vi "Start Measurements Command.vi"(6 "Reply to me":refnum<class "Result Reply Msg.lvclass">, 8 "error in (no error)":errorcluster, 9 "Objects":string[](array[string]), 10 "Controller name":string="Monitor Controller", 11 "Monitor-Pulse in":refnum<class "Monitor-Pulse.lvclass">) -> (0 "error out":errorcluster, 3 "Monitor-Pulse out":refnum<class "Monitor-Pulse.lvclass">)   [LabVIEW 2016, in "Monitor-Pulse.lvclass"]
uses:
  Monitor-Pulse.lvclass
  C:/Program Files/National Instruments/LabVIEW 2016/vi.lib/ActorFramework/Actor/Actor.lvclass
  Measure_core/Template Module Messages/Result Reply Msg/Result Reply Msg.lvclass
  C:/github/Measure_core/Da Base Messages/Self-Addressed Msg/Self-addressed Msg.lvclass
  <vilib>/ActorFramework/Actor/Actor.lvclass/Actor.ctl
  <vilib>/ActorFramework/Message Enqueuer/Message Enqueuer.lvclass/Message Enqueuer.ctl
  Measure_core/Template Module Messages/Self-Addressed Msg/Self-addressed Msg.lvclass/Self-addressed Msg.ctl
  Measure_core/Controllers/Process Controller Messages/Start Measurements Msg/Start Measurements Msg.lvclass/Start Measurements Msg.ctl
  Measure_core/Template Module Messages/Self-Addressed Msg/Write Return Enqueuer.vi
  <vilib>/ActorFramework/Message Enqueuer/Init from Existing Queue.vi
  <vilib>/ActorFramework/Message Enqueuer/Enqueue.vi
  Measure_core/Controllers/Process Controller Messages/Start Measurements Msg/Start Measurements Msg.lvclass
  C:/Program Files/National Instruments/LabVIEW 2016/vi.lib/ActorFramework/Message/Message.lvclass
  <vilib>/ActorFramework/Message Priority Queue/Priority Enqueue.vi
  <vilib>/ActorFramework/Message Enqueuer/Message Enqueuer.lvclass
  <vilib>/ActorFramework/Actor/Actor.lvclass
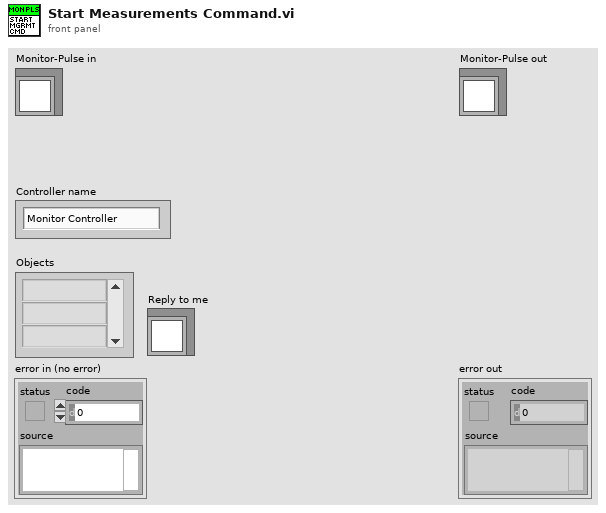
[diagram p1: front panel]
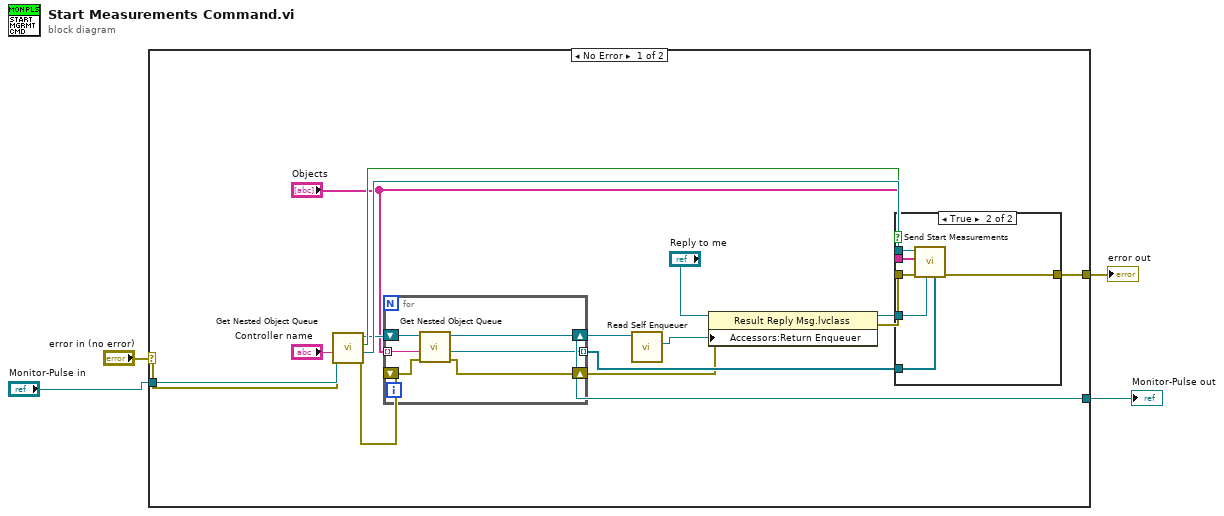
[diagram p0: block diagram]
diagram:
  n1 = case shown="No Error" "error in (no error)" {
    selector: "error in (no error)" -> [w15 w35]
    tunnel: [w17 w35] -> w2
    tunnel: [w5 w34] -> w1
    tunnel: "Monitor-Pulse in" -> [w16 w34]
    frame No Error {
      n2 = call-dynamic "Get Nested Object Queue.vi"("error in (no error)"=w15, "Name"="Controller name", "Measure Object in"=w16) -> ("error out"=w10:errorcluster, "Object Enqueuer"=w19:refnum<class "Message Enqueuer.lvclass">, "Found?"=w18:bool, "Measure Object out"=w11:refnum<class "Monitor-Pulse.lvclass">)  [unwired: 5 in]
      n3 = for {
        tunnel: "Objects" -> [w26] mode=indexing
        shift-right: [w24] -> w5
        shift-left: w11 -> [w25]
        shift-right: [w22] -> w6
        shift-left: w10 -> [w23]
        tunnel: [w21] -> w9 mode=indexing
        n4 = call-dynamic "Get Nested Object Queue.vi"("error in (no error)"=w23, "Name"=w26, "Measure Object in"=w25) -> ("error out"=w22:errorcluster, "Object Enqueuer"=w21:refnum<class "Message Enqueuer.lvclass">, "Measure Object out"=w24:refnum<class "Monitor-Pulse.lvclass">)  [unwired: 5 in, 1 out]
      }
      n5 = call <vilib>:"Read Self Enqueuer.vi"("Actor"=w5) -> ("Self Enqueuer"=w14:refnum<class "Message Enqueuer.lvclass">)  [unwired: 10 in]
      n6 = property class="Result Reply Msg.lvclass"(reference="Reply to me", error in=w6, "Accessors:Return Enqueuer"=w14) -> (reference out=w13:refnum<class "Result Reply Msg.lvclass">, error out=w12:errorcluster)
      n7 = case shown="True" w18 {
        tunnel: w19 -> [_ w33]
        tunnel: w12 -> [w27 w32]
        tunnel: [w27 w31] -> w17
        tunnel: w13 -> [_ w30]
        tunnel: w9 -> [_ w29]
        tunnel: "Objects" -> [_ w28]
        frame False {
        }
        frame True {
          n8 = call "Send Start Measurements.vi"("Objects enqueuers"=w29, "Reply to"=w30, "error in (no error)"=w32, "Objects"=w28, "Message Enqueuer"=w33) -> ("error out"=w31:errorcluster)  [unwired: 5 in, 1 out]
        }
      }
    }
    frame Error {
    }
  }
  "error out" <- w2
  "Monitor-Pulse out" <- w1
